vi "Shooter Controller.vi"(8 "error in":errorcluster) -> ()   [LabVIEW 2020]
doc: "This VI executes continuously carrying out the current operation and responding to updates or new operations. It will often contain the timing or control code that is difficult to place directly in TeleOp. This VI generally opens all sensors and motors and isolates the rest of the robot code from knowing how the operations are carried out."
uses:
  <vilib>/Rock Robotics/WPI/Framework/Completion Status.ctl
  Shooter Setpoints.ctl
  Shooter Operations.ctl
  <vilib>/Rock Robotics/SystemInterfaces/DIO/FPGA_DIOChannel.ctl
  <vilib>/Rock Robotics/WPI/ThirdParty/REV Robotics/REVLib/Typedef/Spark MAX Control Type.ctl
  <vilib>/Rock Robotics/WPI/ThirdParty/Phoenix-LabVIEW/Motor Controller/Controls/CTRE_Phoenix_MotorControl_ControlMode.ctl
  <vilib>/Rock Robotics/WPI/Counter/WPI_CounterDigitalInputToDigitalSource.vi
  <vilib>/Rock Robotics/Network Tables/NT Write Number.vi
  <vilib>/Rock Robotics/WPI/ThirdParty/Phoenix-LabVIEW/Motor Controller/Get/CTRE_Phoenix_MotorController_GetVoltage.vi
  <vilib>/Rock Robotics/Network Tables/NT Write Boolean.vi
panel:
  out "Shooter Ready?":bool
  out "flywheel v":dbl(graph)
  out "Top Flywheel voltage":dbl(graph)
  in  "FeedFwd Value":dbl format="%.2f"
  in  "PID gains":T1={"proportional gain (Kp)"=1.0, "integral time (Ki)"=0.0, "derivative time (Kd)"=0.0} {"derivative time (Kd)" format="%.4e"; "integral time (Ki)" format="%.3f"; "proportional gain (Kp)" format="%.4e"}
  in  "flywheel":T2={"P Gain"=8e-06, "I Gain"=0.0, "D Gain"=0.0005, "F Gain"=0.00019, "I Zone"=0.0, "Min Output"=-1.0, "Max Output"=1.0}
  out "flywheel":T3(graph)
  out "top flywheel":cluster{"top flywheel (vol)":dbl, "Rate":dbl}(graph)
  in  "top flywheel rest (test)":dbl
  in  "flywheel rest (test)":dbl
  in  "Interactive Values":T4
  out "Current\nCmd":string
  in  "Buttons":cluster{"Execute Cmd":bool, "Abort Cmd":bool}
  out "Command Timing":cluster{"Start Time (ms)":u32, "Iterations":i32}
  out "Status":T6
  # "Tip: It may be helpful to observe inputs and sensor values.\nYou may also want to display tuning or debugging controls."
  # "Interactive Command: You may fill in the settings for a command\nand schedule it with the Execute button. You can observe and abort\nany command while fine tuning the code for the controller."
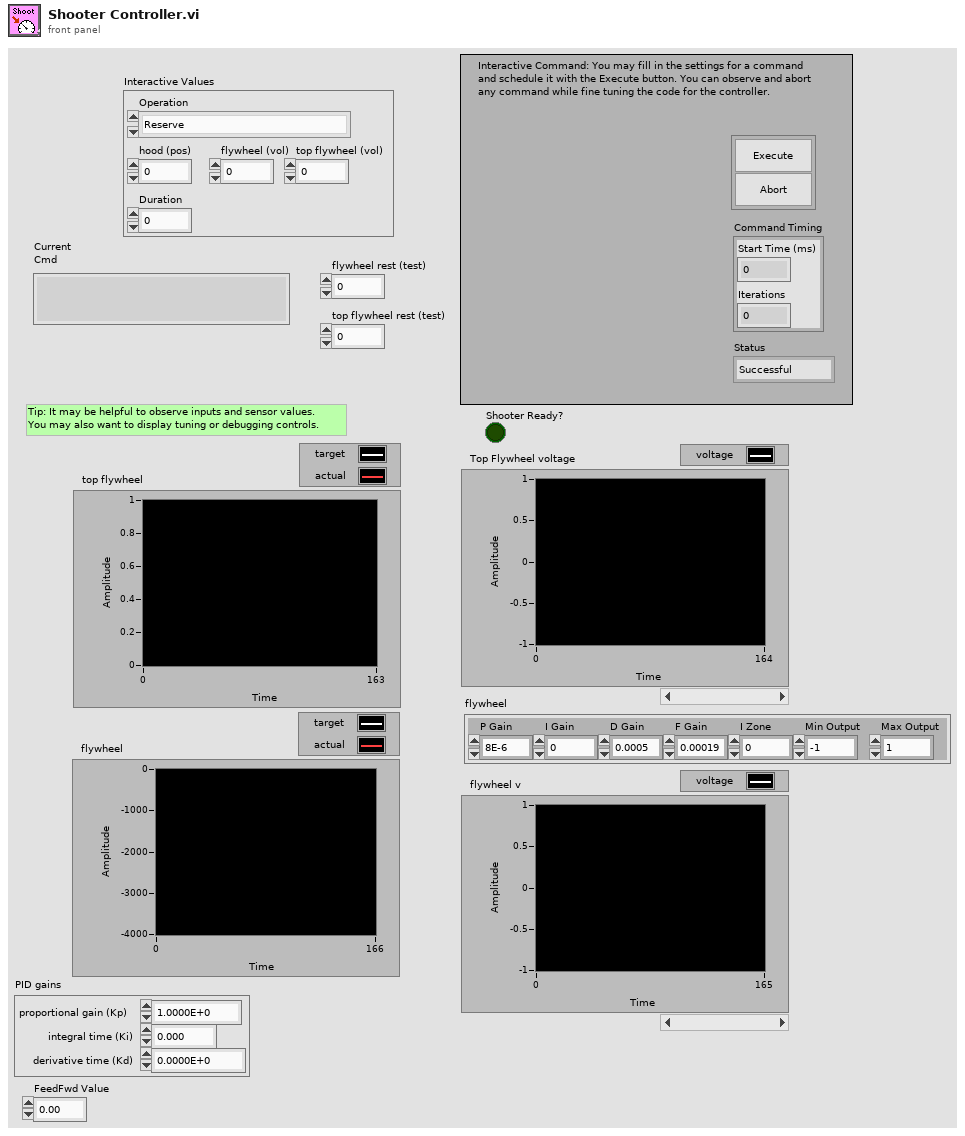
[diagram p1: front panel]
types:
  T1 = cluster{"proportional gain (Kp)":dbl, "integral time (Ki)":dbl, "derivative time (Kd)":dbl}
  T2 = cluster{"P Gain":dbl, "I Gain":dbl, "D Gain":dbl, "F Gain":dbl, "I Zone":dbl, "Min Output":dbl, "Max Output":dbl}
  T3 = cluster{"flywheel (vol)":dbl, "Sensor Velocity":dbl}
  T4 = typedef "Shooter Setpoints.ctl" = cluster{"Operation":T5, "hood (pos)":dbl, "Duration":dbl, "flywheel (vol)":dbl, "top flywheel (vol)":dbl}
  T5 = typedef "Shooter Operations.ctl" = enum16{"Reserve", "Read Current", "Rest", "Immediate"}
  T6 = typedef "Completion Status.ctl" = enum16{"Successful", "Aborted", "Incomplete"}
  T7 = typedef "FPGA_DIOChannel.ctl" = enum8{"DIO 0", "DIO 1", "DIO 2", "DIO 3", "DIO 4", "DIO 5", "DIO 6", "DIO 7", "DIO 8", "DIO 9", "DIO MXP 0", "DIO MXP 1", "DIO MXP 2", "DIO MXP 3", "DIO MXP 4", "DIO MXP 5", "DIO MXP 6", "DIO MXP 7", "DIO MXP 8", "DIO MXP 9", "DIO MXP 10", "DIO MXP 11", "DIO MXP 12", "DIO MXP 13", "DIO MXP 14", "DIO MXP 15", "SPI Port CS1", "SPI Port CS2", "SPI Port CS3", "SPI Port MISO", "SPI Port MOSI", "Invalid"}
  T8 = cluster{"P Gain":dbl, "I Gain":dbl, "D Gain":dbl, "F Gain":dbl, "I Zone":dbl}
  T9 = typedef "WPI_MotorControlDeviceRef.ctl" = cluster{"DeviceStatus":errorcluster, "Type":T10, "PWM":cluster{"PWM Channel":T11, "DeadBand":T12}, "CAN":cluster{"Device Number":u8, "SetOutput VI Ref":variant, "GetOutput VI Ref":variant, "Enable VI Ref":variant, "Disable VI Ref":variant, "Data":variant}, "Invert":bool, "DIO PWM":cluster{"PWM \"Enable\" Channel":T11, "DIOChannel":T7, "PWM Rate":dbl}}
  T10 = typedef "WPI_MotorControlType.ctl" = enum16{"PWM", "CAN", "DIO PWM"}
  T11 = typedef "FPGA_DIOPWMChannel.ctl" = enum8{"PWM 0", "PWM 1", "PWM 2", "PWM 3", "PWM 4", "PWM 5", "PWM 6", "PWM 7", "PWM 8", "PWM 9", "PWM MXP 0", "PWM MXP 1", "PWM MXP 2", "PWM MXP 3", "PWM MXP 4", "PWM MXP 5", "PWM MXP 6", "PWM MXP 7", "PWM MXP 8", "PWM MXP 9", "Invalid"}
  T12 = typedef "WPI_PWMDeadband.ctl" = cluster{"Name":string, "maxPositivePwm":i32, "minPositivePwm":i32, "centerPwm":i32, "maxNegativePwm":i32, "minNegativePwm":i32, "angularRange":u16}
  T13 = typedef "WPI_DigitalInputDevRef.ctl" = cluster{"DevStatus":errorcluster, "DIO Channel":T7}
  T14 = typedef "FPGA_CounterEncoderSourceConvertionLVSourceType.ctl" = cluster{"DevStatus":errorcluster, "AnalogTriggerMode?":bool, "DigitalMode":cluster{"DIO Channel":T15}, "AnalogTriggerMode":cluster{"AnalogTriggerIndex":T16, "OutputType":T17}}
  T15 = typedef "FPGA_DIODigitalSourceChannel.ctl" = enum8{"DIO 0", "DIO 1", "DIO 2", "DIO 3", "DIO 4", "DIO 5", "DIO 6", "DIO 7", "DIO 8", "DIO 9", "DIO MXP 0", "DIO MXP 1", "DIO MXP 2", "DIO MXP 3", "DIO MXP 4", "DIO MXP 5", "DIO MXP 6", "DIO MXP 7", "DIO MXP 8", "DIO MXP 9", "DIO MXP 10", "DIO MXP 11", "DIO MXP 12", "DIO MXP 13", "DIO MXP 14", "DIO MXP 15", "SPI Port CS1", "SPI Port CS2", "SPI Port CS3", "SPI Port MISO", "SPI Port MOSI", "Disabled"}
  T16 = typedef "FPGA_AnalogTriggerIndex.ctl" = enum8{"Trig 0", "Trig 1", "Trig 2", "Trig 3", "Trig 4", "Trig 5", "Trig 6", "Trig 7", "Invalid"}
  T17 = typedef "FPGA_AnalogTriggerOutType.ctl" = enum16{"InWindow", "TriggerState", "Rising", "Falling"}
  T18 = typedef "WPI_EncoderDevRef.ctl" = cluster{"DevStatus":errorcluster, "EncoderIndex":T19, "CounterIndex":T20, "DistancePerCount":dbl, "Decoding Type":T21}
  T19 = typedef "FPGA_EncoderIdx.ctl" = enum8{"Enc 0", "Enc 1", "Enc 2", "Enc 3", "Enc 4", "Enc 5", "Enc 6", "Enc 7", "Invalid"}
  T20 = typedef "FPGA_CounterCtrSystemIndex.ctl" = enum8{"Ctr 0", "Ctr 1", "Ctr 2", "Ctr 3", "Ctr 4", "Ctr 5", "Ctr 6", "Ctr 7", "Invalid"}
  T21 = typedef "WPI_EncoderType.ctl" = enum16{"1x", "2x", "4x"}
  T22 = typedef "Command Status Info.ctl" = cluster{"Name":string, "Status":T6, "notifier out":T23}
  T23 = typedef "Completion Notifier.ctl" = refnum<notifier>
  T24 = cluster{"Current Command":T4, "Command Timing":cluster{"Start Time (ms)":u32, "Iterations":i32}, "Command Arguments":cluster{"Command Info":T22, "Description":string, "Default Command":T4, "queue out":refnum<queue>, "Subsystem Name":string}}
  T25 = typedef "Spark MAX Control Type.ctl" = enum16{"Percent VBus", "Voltage", "Velocity", "Position", "Smart Motion", "Current", "Smart Velocity"}
  T26 = typedef "CTRE_Phoenix_MotorControl_ControlMode.ctl" = u16
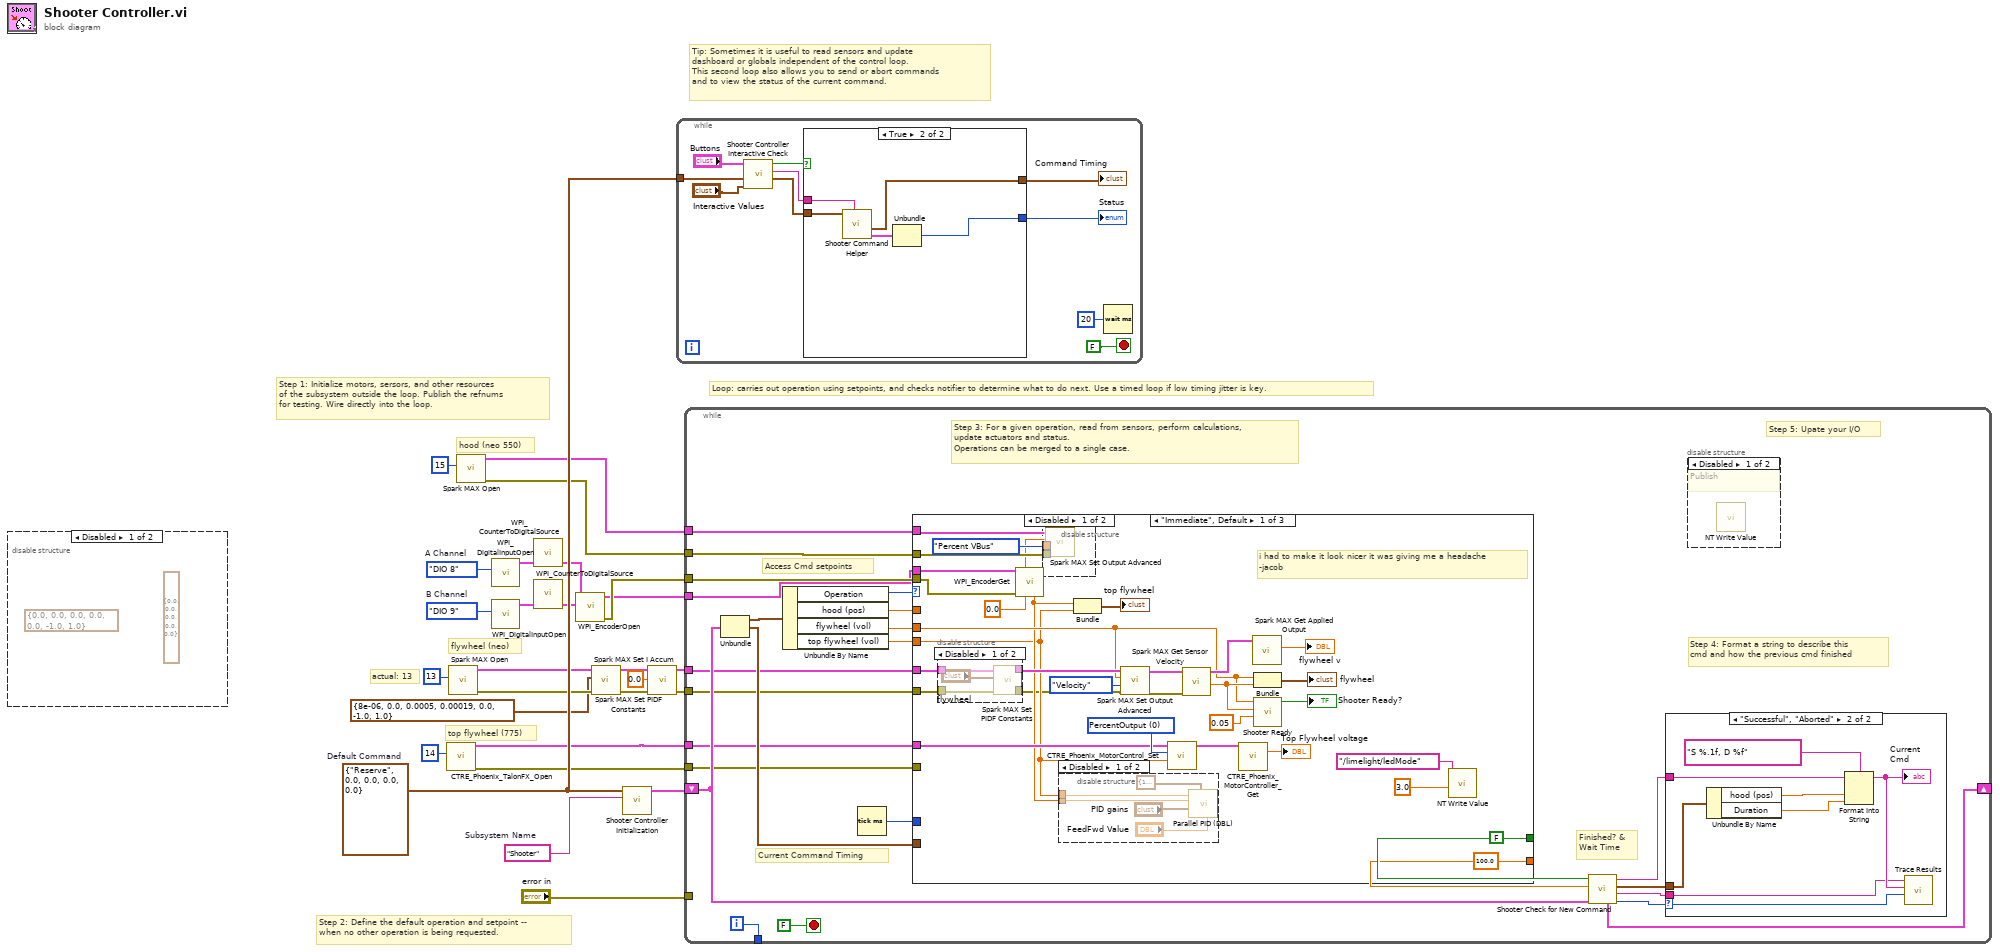
[diagram p0: block diagram]
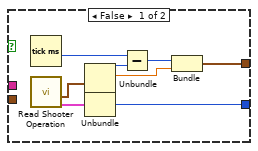
[diagram p3: hidden frame]
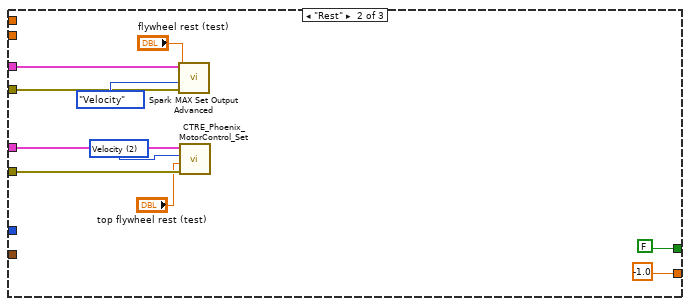
[diagram p9: hidden frame]
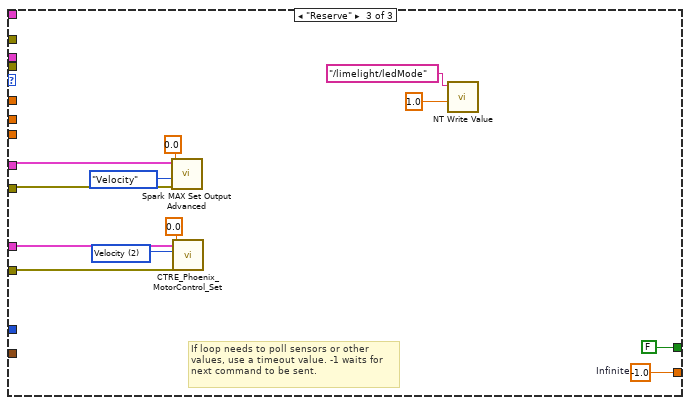
[diagram p10: hidden frame]
diagram:
  w9 = FPGA_DIOChannel."DIO 9"  # B Channel
  w8 = FPGA_DIOChannel."DIO 8"  # A Channel
  w24 = T4 {"Operation"=enum."Reserve", "hood (pos)"=0.0, "Duration"=0.0, "flywheel (vol)"=0.0, "top flywheel (vol)"=0.0}  # Default Command
  w25 = "Shooter"  # Subsystem Name
  # "actual: 13"
  # "flywheel (neo)"
  # "hood (neo 550)"
  # "top flywheel (775)"
  # "Tip: Sometimes it is useful to read sensors and update\ndashboard or globals independent of the control loop.\nThis second loop also allows you to send or abort commands\nand to view the status of the current command."
  # "Step 2: Define the default operation and setpoint --\nwhen no other operation is being requested."
  # "Step 1: Initialize motors, sersors, and other resources\nof the subsystem outside the loop. Publish the refnums\nfor testing. Wire directly into the loop."
  # "Loop: carries out operation using setpoints, and checks notifier to determine what to do next. Use a timed loop if low timing jitter is key."
  n1 = disable-structure shown="Disabled" {
    frame Disabled {
      (unwired) T2 {"P Gain"=0.0, "I Gain"=0.0, "D Gain"=0.0, "F Gain"=0.0, "I Zone"=0.0, "Min Output"=-1.0, "Max Output"=1.0} ("Flywheel PID")
      (unwired) T8 {"P Gain"=0.0, "I Gain"=0.0, "D Gain"=0.0, "F Gain"=0.0, "I Zone"=0.0} ("Top Flywheel PID")
    }
    frame Enabled {
    }
  }
  n2 = call <vilib>:"CTRE_Phoenix_TalonFX_Open.vi"("Device Number"=u8 14) -> ("error out"=w2:errorcluster, "PhoenixMotorControlDevRef"=w3:T9)  [unwired: 9 in]
  n3 = call <vilib>:"Spark MAX Open.vi"("Device Number"=u8 13) -> ("error out"=w18:errorcluster, "MotorControlDeviceRef"=w19:T9)  [unwired: 9 in]
  n4 = call <vilib>:"Spark MAX Open.vi"("Device Number"=u8 15) -> ("error out"=w23:errorcluster, "MotorControlDeviceRef"=w22:T9)  [unwired: 9 in]
  n5 = call <vilib>:"WPI_DigitalInputOpen.vi"("DIO Channel"=w8) -> ("DigitalInputDevRef"=w6:T13)  [unwired: 1 in, 9 out]
  n6 = call <vilib>:"WPI_DigitalInputOpen.vi"("DIO Channel"=w9) -> ("DigitalInputDevRef"=w7:T13)  [unwired: 1 in, 9 out]
  n7 = call-poly <vilib>:"WPI_CounterToDigitalSource.vi"("DigitalInputDevRef"=w6) -> ("Digital Source"=w10:T14)  [unwired: 6 out]
  n8 = call-poly <vilib>:"WPI_CounterToDigitalSource.vi"("DigitalInputDevRef"=w7) -> ("Digital Source"=w11:T14)  [unwired: 6 out]
  n9 = call <vilib>:"WPI_EncoderOpen.vi"("BSource"=w11, "ASource"=w10) -> ("error out"=w5:errorcluster, "EncoderDevRef"=w4:T18)  [unwired: 8 in]
  n10 = call <vilib>:"Spark MAX Set PIDF Constants.vi"("error in"=w18, "PID Constants"=T2 {"P Gain"=8e-06, "I Gain"=0.0, "D Gain"=0.0005, "F Gain"=0.00019, "I Zone"=0.0, "Min Output"=-1.0, "Max Output"=1.0} ("flywheel 2"), "MotorControlDeviceRef"=w19) -> ("error out"=w14:errorcluster, "MotorControlDeviceRef"=w16:T9)  [unwired: 7 in]
  n11 = call "Shooter Controller Initialization.vi"("Subsystem Name"=w25, "Default Command"=w24) -> ("Current Command"=w26:T24)  [unwired: 9 in]
  n12 = call <vilib>:"Spark MAX Set I Accum.vi"("error in"=w14, "I Accum"=0.0, "MotorControlDeviceRef"=w16) -> ("error out"=w13:errorcluster, "MotorControlDeviceRef"=w15:T9)  [unwired: 7 in]
  n13 = while {
    tunnel: w24 -> [w34]
    stop <- FALSE stop-if-true
    n14 = call "Shooter Controller Interactive Check.vi"("Interactive Command in"="Interactive Values", "Default Command"=w34, "Buttons"="Buttons") -> ("Interactive Command out"=w31:T4, "Trace String"=w32:string, "Schedule"=w33:bool)  [unwired: 6 in]
    n15 = case shown="True" w33 {
      tunnel: [w45 w50] -> w30
      tunnel: w31 -> [_ w48]
      tunnel: [w41 w46] -> w29
      tunnel: w32 -> [_ w49]
      frame False {
        n16 = Tick Count (ms)() -> (millisecond timer value=w40:u32)
        n17 = call "Read Shooter Operation.vi"() -> ("Command Info"=w38:T22, "SubSystem Data"=w39:T4)  [unwired: 9 in, 1 out]
        n18 = Unbundle(w39) -> ("Operation"=w44:T5, "hood (pos)"=w42:dbl)  [unwired: 3 out]
        n19 = Unbundle(w38) -> ("Status"=w45:T6)  [unwired: 2 out]
        n20 = Subtract(x=w40, y=w44) -> (x-y=w43:u32)
        n21 = Bundle(w43, "hood (pos)"=w42) -> (w41:cluster{u32, "hood (pos)":dbl})  [unwired: 1 in]
      }
      frame True {
        n22 = call "Shooter Command Helper.vi"("Description"=w49, "SubSystem Data"=w48) -> ("Command Info Out"=w47:T22, "Command Timing"=w46:cluster{"Start Time (ms)":u32, "Iterations":i32})  [unwired: 7 in, 1 out]
        n23 = Unbundle(w47) -> ("Status"=w50:T6)  [unwired: 2 out]
      }
    }
    "Status" <- w30
    "Command Timing" <- w29
    n24 = Wait (ms)(milliseconds to wait=u32 20) -> ()  [unwired: 1 out]
  }
  n25 = while {
    shift-right: [w67] -> _
    shift-left: w26 -> [w60]
    tunnel: [w74] -> _
    tunnel: "error in" -> [_]
    tunnel: w23 -> [w59]
    tunnel: w22 -> [w58]
    tunnel: w15 -> [w57]
    tunnel: w2 -> [w56]
    tunnel: w3 -> [w55]
    tunnel: w13 -> [w53]
    tunnel: w5 -> [w52]
    tunnel: w4 -> [w51]
    i -> [w74]
    stop <- FALSE stop-if-true
    # "Step 5: Upate your I/O"
    # "Step 4: Format a string to describe this\ncmd and how the previous cmd finished"
    # "Current Command Timing"
    # "Access Cmd setpoints"
    # "Finished? &\nWait Time"
    # "Step 3: For a given operation, read from sensors, perform calculations,\nupdate actuators and status.\nOperations can be merged to a single case."
    n26 = Unbundle(w60) -> ("Current Command"=w73:T4, "Command Timing"=w69:cluster{"Start Time (ms)":u32, "Iterations":i32})  [unwired: 1 out]
    n27 = Unbundle By Name(w73) -> ("Operation"=w72:T5, "hood (pos)"=w71:dbl, "flywheel (vol)"=w68:dbl, "top flywheel (vol)"=w54:dbl)
    n28 = Tick Count (ms)() -> (millisecond timer value=w70:u32)
    n29 = case shown="\"Immediate\", Default" w72 {
      tunnel: [100.0 -1.0 ("Infinite") w152] -> w65
      tunnel: [FALSE ("ignore previous (F)") FALSE ("ignore previous (F)") FALSE ("ignore previous (F)")] -> w66
      tunnel: w69 -> [_ _ _]
      tunnel: w71 -> [_ _ _]
      tunnel: w70 -> [_ _ _]
      tunnel: w68 -> [w92 _ _]
      tunnel: w59 -> [w113 _ _]
      tunnel: w58 -> [w112 _ _]
      tunnel: w53 -> [w89 w137 w145]
      tunnel: w57 -> [w110 w138 w146]
      tunnel: w56 -> [_ w136 w143]
      tunnel: w55 -> [w100 w135 w144]
      tunnel: w54 -> [w90 _ _]
      tunnel: w52 -> [w104 _ _]
      tunnel: w51 -> [w103 _ _]
      frame "Immediate", Default {
        w101 = T26 0 items=["PercentOutput"=0, "Position"=1, "Velocity"=2, "Current"=3, "Follower"=5, "MotionProfile"=6, "MotionMagic"=7, "MotionProfileArc"=10, "Disabled"=15] ("Control Mode")
        # "i had to make it look nicer it was giving me a headache\n-jacob"
        n30 = disable-structure shown="Disabled" {
          disable-tunnel: w110 -> [w123 w125]
          disable-tunnel: [w122 w125] -> w109
          disable-tunnel: w89 -> [w120 w124]
          disable-tunnel: [w119 w124] -> w88
          frame Disabled {
            n31 = call <vilib>:"Spark MAX Set PIDF Constants.vi"("error in"=w120, "PID Constants"="flywheel", "MotorControlDeviceRef"=w123) -> ("error out"=w119:errorcluster, "MotorControlDeviceRef"=w122:T9)  [unwired: 7 in]
          }
          frame Enabled {
          }
        }
        n32 = call <vilib>:"WPI_EncoderGet.vi"("error in (no error)"=w104, "EncoderDevRef"=w103) -> ("Rate"=w91:dbl)  [unwired: 4 in, 5 out]
        n33 = disable-structure shown="Disabled" {
          disable-tunnel: w113 -> [w118 _]
          disable-tunnel: w112 -> [w117 _]
          disable-tunnel: Spark_MAX_Control_Type."Percent VBus" ("Control Mode") -> [w116 _]
          disable-tunnel: 0.0 ("Setpoint") -> [w115 _]
          frame Disabled {
            n34 = call <vilib>:"Spark MAX Set Output Advanced.vi"("error in (no error)"=w118, "Control Mode"=w116, "Setpoint"=w115, "MotorControlDevRef"=w117) -> ()  [unwired: 6 in, 2 out]
          }
          frame Enabled {
          }
        }
        n35 = disable-structure shown="Disabled" {
          disable-tunnel: w91 -> [w127 _]
          disable-tunnel: w90 -> [w126 _]
          frame Disabled {
            n36 = call <vilib>:"Parallel PID (DBL).vi"("FeedFwd Value"="FeedFwd Value", "output range"=cluster{"high":dbl, "low":dbl} {"high"=1.0, "low"=-1.0}, "PID gains"="PID gains", "process variable"=w127, "setpoint"=w126) -> ()  [unwired: 3 in, 4 out]
          }
          frame Enabled {
          }
        }
        n37 = Bundle("Rate"=w91, "top flywheel (vol)"=w90) -> (→"top flywheel":cluster{"Rate":dbl, "top flywheel (vol)":dbl})  [unwired: 1 in]
        n38 = call <vilib>:"Spark MAX Set Output Advanced.vi"("error in (no error)"=w88, "Control Mode"=Spark_MAX_Control_Type."Velocity", "Setpoint"=w92, "MotorControlDevRef"=w109) -> ("error out"=w106:errorcluster, "MotorControlDevRef"=w98:T9)  [unwired: 6 in]
        n39 = call <vilib>:"CTRE_Phoenix_MotorControl_Set.vi"("Output"=w90, "Control Mode"=w101, "PhoenixMotorControlDevRef"=w100) -> ("PhoenixMotorControlDevRef"=w94:T9)  [unwired: 7 in, 1 out]
        n40 = call <vilib>:"Spark MAX Get Sensor Velocity.vi"("error in (no error)"=w106, "MotorControlDevRef in"=w98) -> ("Sensor Velocity"=w93:dbl, "MotorControlDevRef out"=w95:T9)  [unwired: 6 in, 2 out]
        n41 = call-poly <vilib>:"CTRE_Phoenix_MotorController_Get.vi"("PhoenixMotorControlDevRef"=w94) -> ("Percent Output"=→"Top Flywheel voltage":dbl)  [unwired: 10 in, 4 out]
        n42 = call <vilib>:"Spark MAX Get Applied Output.vi"("MotorControlDevRef in"=w95) -> ("Applied Output"=→"flywheel v":dbl)  [unwired: 7 in, 3 out]
        n43 = Bundle("flywheel (vol)"=w92, "Sensor Velocity"=w93) -> (→"flywheel":T3)  [unwired: 1 in]
        n44 = call "Shooter Ready.vi"("percent err"=0.05, "flywheel speed"=w93, "target speed"=w92) -> ("up to speed?"=→"Shooter Ready?":bool)  [unwired: 8 in]
        n45 = call-poly <vilib>:"NT Write Value.vi"("Numeric"=3.0, "Name"="/limelight/ledMode") -> ()  [unwired: 9 in, 1 out]
      }
      frame "Rest" {
        w139 = T26 2 items=["PercentOutput"=0, "Position"=1, "Velocity"=2, "Current"=3, "Follower"=5, "MotionProfile"=6, "MotionMagic"=7, "MotionProfileArc"=10, "Disabled"=15] ("Control Mode")
        n46 = call <vilib>:"Spark MAX Set Output Advanced.vi"("error in (no error)"=w137, "Control Mode"=Spark_MAX_Control_Type."Velocity", "Setpoint"="flywheel rest (test)", "MotorControlDevRef"=w138) -> ()  [unwired: 6 in, 2 out]
        n47 = call <vilib>:"CTRE_Phoenix_MotorControl_Set.vi"("error in (no error)"=w136, "Output"="top flywheel rest (test)", "Control Mode"=w139, "PhoenixMotorControlDevRef"=w135) -> ()  [unwired: 6 in, 2 out]
      }
      frame "Reserve" {
        w149 = T26 2 items=["PercentOutput"=0, "Position"=1, "Velocity"=2, "Current"=3, "Follower"=5, "MotionProfile"=6, "MotionMagic"=7, "MotionProfileArc"=10, "Disabled"=15] ("Control Mode")
        w152 = -1.0  # Infinite
        # "If loop needs to poll sensors or other\nvalues, use a timeout value. -1 waits for\nnext command to be sent."
        n48 = call <vilib>:"Spark MAX Set Output Advanced.vi"("error in (no error)"=w145, "Control Mode"=Spark_MAX_Control_Type."Velocity", "Setpoint"=0.0, "MotorControlDevRef"=w146) -> ()  [unwired: 6 in, 2 out]
        n49 = call <vilib>:"CTRE_Phoenix_MotorControl_Set.vi"("error in (no error)"=w143, "Output"=0.0, "Control Mode"=w149, "PhoenixMotorControlDevRef"=w144) -> ()  [unwired: 6 in, 2 out]
        n50 = call-poly <vilib>:"NT Write Value.vi"("Numeric"=1.0, "Name"="/limelight/ledMode") -> ()  [unwired: 9 in, 1 out]
      }
    }
    n51 = call "Shooter Check for New Command.vi"("Current Command"=w60, "Wait time (ms)"=w65, "Finished?"=w66) -> ("Completion"=w61:T6, "Subsystem Name"=w62:string, "Current Command"=w63:T4, "Initial Trace String"=w64:string, "NextCommand"=w67:T24)  [unwired: 4 in]
    n52 = case shown="\"Successful\", \"Aborted\"" w61 {
      selector: w61 -> [_ w83]
      tunnel: w64 -> [_ w79]
      tunnel: w63 -> [_ w80]
      tunnel: w62 -> [_ w76]
      frame "Incomplete", Default {
        # "Continuing current command"
      }
      frame "Successful", "Aborted" {
        # "Report and setup for next command"
        n53 = Unbundle By Name(w80) -> ("hood (pos)"=w82:dbl, "Duration"=w77:dbl)
        n54 = Format Into String(format string="S %.1f, D %f", initial string=w79, w82, w77) -> (resulting string=w78:string)  [unwired: 1 in, 1 out]
        "Current\nCmd" <- w78
        n55 = call <vilib>:"Trace Results.vi"("Status of previous command"=w83, "Description"=w78, "Subsystem"=w76) -> ()  [unwired: 9 in]
      }
    }
    n56 = disable-structure shown="Disabled" {
      frame Disabled {
        # "Publish"
        n57 = call-poly <vilib>:"NT Write Value.vi"() -> ()  [unwired: 11 in, 1 out]
      }
      frame Enabled {
      }
    }
  }
